vi "Main.vi"() -> ()   [LabVIEW 2013]
uses:
  Ch.ctl
panel:
  out "10 x 10":bool[][](array[boolean])
  in  "Exit":bool
  in  "Stop":bool
  in  "X":bool
  in  "Y":bool
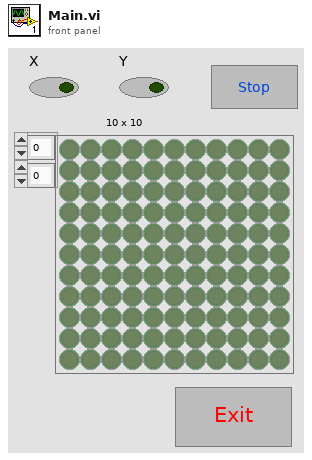
[diagram p1: front panel]
types:
  T1 = typedef "Ch.ctl" = enum16{"X", "Y", "Stop", "IntY", "IntX", "Init", "Exit"}
  T2 = enum32{"Invalid", "Standard", "Closed", "Hidden", "Minimized", "Maximized"}
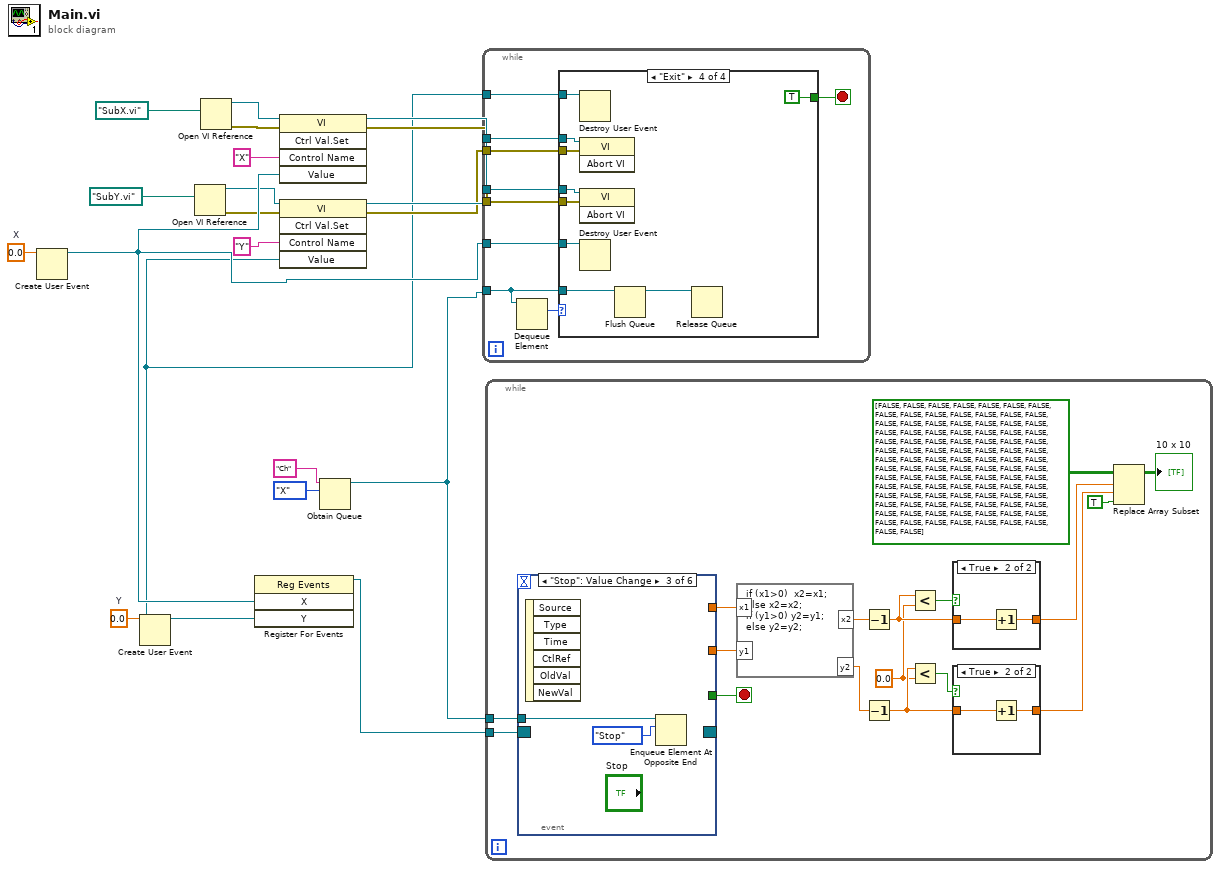
[diagram p0: block diagram]
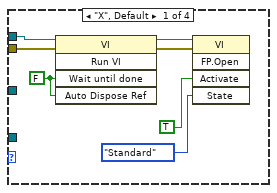
[diagram p2: hidden frame]
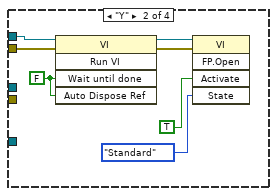
[diagram p3: hidden frame]
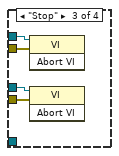
[diagram p4: hidden frame]
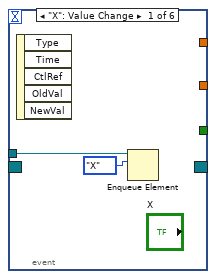
[diagram p7: hidden frame]
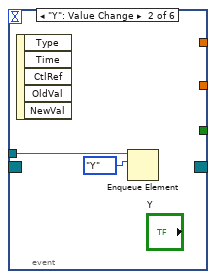
[diagram p8: hidden frame]
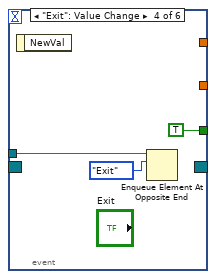
[diagram p9: hidden frame]
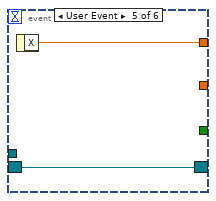
[diagram p10: hidden frame]
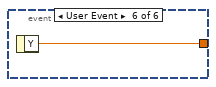
[diagram p11: hidden frame]
diagram:
  w15 = 0.0  # Y
  w17 = 0.0  # X
  n1 = Create User Event(user event datatype=w17) -> (user event=w10:refnum<user-event>)  [unwired: 1 in, 1 out]
  n2 = Create User Event(user event datatype=w15) -> (user event=w1:refnum<user-event>)  [unwired: 1 in, 1 out]
  n3 = Open VI Reference(vi path=path "SubY.vi") -> (vi reference=w7:refnum<vi>, error out=w6:errorcluster)  [unwired: 5 in]
  n4 = Open VI Reference(vi path=path "SubX.vi") -> (vi reference=w14:refnum<vi>, error out=w13:errorcluster)  [unwired: 5 in]
  n5 = register-events(w10, w1) -> (reference out=w16:refnum<event-registration>)  [unwired: 2 in, 1 out]
  n6 = invoke class="VI" method="Ctrl Val.Set"(reference=w14, error in=w13, "Control Name"="X", "Value"=w10) -> (reference out=w9:refnum<vi>, error out=w8:errorcluster)  [unwired: 1 in, 3 out]
  n7 = invoke class="VI" method="Ctrl Val.Set"(reference=w7, error in=w6, "Control Name"="Y", "Value"=w1) -> (reference out=w3:refnum<vi>, error out=w2:errorcluster)  [unwired: 1 in, 3 out]
  n8 = Obtain Queue(name (unnamed)="Ch", element data type=Ch."X" ("Enum")) -> (queue out=w18:refnum<queue>)  [unwired: 3 in, 2 out]
  n9 = while {
    tunnel: w18 -> [w27]
    tunnel: w10 -> [w25]
    tunnel: w1 -> [w26]
    tunnel: w9 -> [w24]
    tunnel: w8 -> [w23]
    tunnel: w3 -> [w22]
    tunnel: w2 -> [w21]
    stop <- w28 stop-if-true
    n10 = Dequeue Element(queue=w27) -> (element=w29:T1)  [unwired: 2 in, 3 out]
    n11 = case shown="\"Exit\"" w29 {
      tunnel: [_ _ _ TRUE ("Wait Until Done")] -> w28
      tunnel: w27 -> [_ _ _ w55]
      tunnel: w26 -> [_ _ _ w53]
      tunnel: w25 -> [_ _ _ w52]
      tunnel: w24 -> [w31 _ w47 w51]
      tunnel: w23 -> [w30 _ w46 w50]
      tunnel: w22 -> [_ w38 w45 w49]
      tunnel: w21 -> [_ w37 w44 w48]
      frame "X", Default {
        w36 = FALSE ("Wait Until Done")
        n12 = invoke class="VI" method="Run VI"(reference=w31, error in=w30, "Wait until done"=w36, "Auto Dispose Ref"=w36) -> (reference out=w35:refnum<vi>, error out=w34:errorcluster)  [unwired: 1 in, 3 out]
        n13 = invoke class="VI" method="FP.Open"(reference=w35, error in=w34, "Activate"=TRUE ("Activate?"), "State"=T2."Standard") -> ()  [unwired: 1 in, 5 out]
      }
      frame "Y" {
        w43 = FALSE ("Wait Until Done")
        n14 = invoke class="VI" method="Run VI"(reference=w38, error in=w37, "Wait until done"=w43, "Auto Dispose Ref"=w43) -> (reference out=w42:refnum<vi>, error out=w41:errorcluster)  [unwired: 1 in, 3 out]
        n15 = invoke class="VI" method="FP.Open"(reference=w42, error in=w41, "Activate"=TRUE ("Activate?"), "State"=T2."Standard") -> ()  [unwired: 1 in, 5 out]
      }
      frame "Stop" {
        n16 = invoke class="VI" method="Abort VI"(reference=w45, error in=w44) -> ()  [unwired: 1 in, 3 out]
        n17 = invoke class="VI" method="Abort VI"(reference=w47, error in=w46) -> ()  [unwired: 1 in, 3 out]
      }
      frame "Exit" {
        n18 = Destroy User Event(user event=w53) -> ()  [unwired: 1 in, 1 out]
        n19 = invoke class="VI" method="Abort VI"(reference=w49, error in=w48) -> ()  [unwired: 1 in, 3 out]
        n20 = invoke class="VI" method="Abort VI"(reference=w51, error in=w50) -> ()  [unwired: 1 in, 3 out]
        n21 = Destroy User Event(user event=w52) -> ()  [unwired: 1 in, 1 out]
        n22 = Flush Queue(queue=w55) -> (queue out=w54:refnum<queue>)  [unwired: 1 in, 2 out]
        n23 = Release Queue(queue=w54) -> ()  [unwired: 2 in, 3 out]
      }
    }
  }
  n24 = while {
    tunnel: w18 -> [w73]
    tunnel: w16 -> [w72]
    stop <- w71 stop-if-true
    w57 = 0.0 ("y")
    n25 = event shown="[2] \"Stop\": Value Change" {
      selector: w72 -> [_ _ _ _ w89 _]
      dyn-events: [_ _ _ _ w89 _] -> _
      timeout: _ -> [_ _ _ _ _ _]
      tunnel: w73 -> [w80 w82 w84 w87 _ _]
      tunnel: [_ _ _ TRUE ("Wait Until Done") _ _] -> w71
      tunnel: [_ _ _ _ w90 _] -> w67
      tunnel: [_ _ _ _ _ w91] -> w66
      event "X": Value Change {
        n26 = event-data() -> ()  [unwired: 1 in, 5 out]
        n27 = Enqueue Element(queue=w80, element=Ch."X" ("Enum")) -> ()  [unwired: 2 in, 3 out]
      }
      event "Y": Value Change {
        n28 = event-data() -> ()  [unwired: 1 in, 5 out]
        n29 = Enqueue Element(queue=w82, element=Ch."Y" ("Enum")) -> ()  [unwired: 2 in, 3 out]
      }
      event "Stop": Value Change {
        n30 = event-data() -> ()  [unwired: 1 in, 6 out]
        n31 = Enqueue Element At Opposite End(queue=w84, element=Ch."Stop" ("Enum")) -> ()  [unwired: 2 in, 3 out]
      }
      event "Exit": Value Change {
        n32 = event-data() -> ()  [unwired: 1 in, 1 out]
        n33 = Enqueue Element At Opposite End(queue=w87, element=Ch."Exit" ("Enum")) -> ()  [unwired: 2 in, 3 out]
      }
      event User Event {
        n34 = event-data() -> ("X"=w90:dbl)  [unwired: 1 in]
      }
      event User Event {
        n35 = event-data() -> ("Y"=w91:dbl)  [unwired: 1 in]
      }
    }
    n36 = formula code="if (x1>0)  x2=x1;\nelse x2=x2;\nif (y1>0) y2=y1;\nelse y2=y2;"("x1"=w67, "y1"=w66) -> ("x2"=w64:dbl, "y2"=w65:dbl)
    n37 = Decrement(x=w64) -> (x-1=w62:dbl)
    n38 = Decrement(x=w65) -> (x-1=w58:dbl)
    n39 = Less?(x=w62, y=w57) -> (x < y?=w63:bool)
    n40 = Less?(x=w58, y=w57) -> (x < y?=w60:bool)
    n41 = case shown="True" w63 {
      tunnel: w62 -> [w77 w79]
      tunnel: [w77 w78] -> w61
      frame False {
      }
      frame True {
        n42 = Increment(x=w79) -> (x+1=w78:dbl)
      }
    }
    n43 = case shown="True" w60 {
      tunnel: w58 -> [w74 w76]
      tunnel: [w74 w75] -> w59
      frame False {
      }
      frame True {
        n44 = Increment(x=w76) -> (x+1=w75:dbl)
      }
    }
    n45 = Replace Array Subset(array=bool[][] [[FALSE, FALSE, FALSE, FALSE, FALSE, FALSE, FALSE, FALSE, FALSE, FALSE], [FALSE, FALSE, FALSE, FALSE, FALSE, FALSE, FALSE, FALSE, FALSE, FALSE], [FALSE, FALSE, FALSE, FALSE, FALSE, FALSE, FALSE, FALSE, FALSE, FALSE], [FALSE, FALSE, FALSE, FALSE, FALSE, FALSE, FALSE, FALSE, FALSE, FALSE], [FALSE, FALSE, FALSE, FALSE, FALSE, FALSE, FALSE, FALSE, FALSE, FALSE], [FALSE, FALSE, FALSE, FALSE, FALSE, FALSE, FALSE, FALSE, FALSE, FALSE], [FALSE, FALSE, FALSE, FALSE, FALSE, FALSE, FALSE, FALSE, FALSE, FALSE], [FALSE, FALSE, FALSE, FALSE, FALSE, FALSE, FALSE, FALSE, FALSE, FALSE], [FALSE, FALSE, FALSE, FALSE, FALSE, FALSE, FALSE, FALSE, FALSE, FALSE], [FALSE, FALSE, FALSE, FALSE, FALSE, FALSE, FALSE, FALSE, FALSE, FALSE]] ("Array"), new element=TRUE, index (row)=w61, index (col)=w59) -> (→"10 x 10":bool[][])
  }
